vi "Drive Controller.vi"(8 "error in":errorcluster) -> ()   [LabVIEW 2017]
doc: "This VI executes continuously carrying out the current operation and responding to updates or new operation requests. It will often contain the timing or control code that is difficult to place directly in TeleOp. This VI generally opens all sensors and motors and isolates the rest of the robot code from knowing implementation details of how the operations are carried out."
uses:
  Drive Setpoints.ctl
  Drive Operations.ctl
  <vilib>/Rock Robotics/WPI/SafetyOutput/WPI_SafetyOutputConfigMenu.ctl
panel:
  out "error out":errorcluster
  in  "Control P":dbl=0.5
  out "Setpoints":T1(graph)
  out "Current\nCmd":string
  # "Tip: It may be helpful to observe inputs and sensor values.\nYou may also want to display tuning or debugging controls."
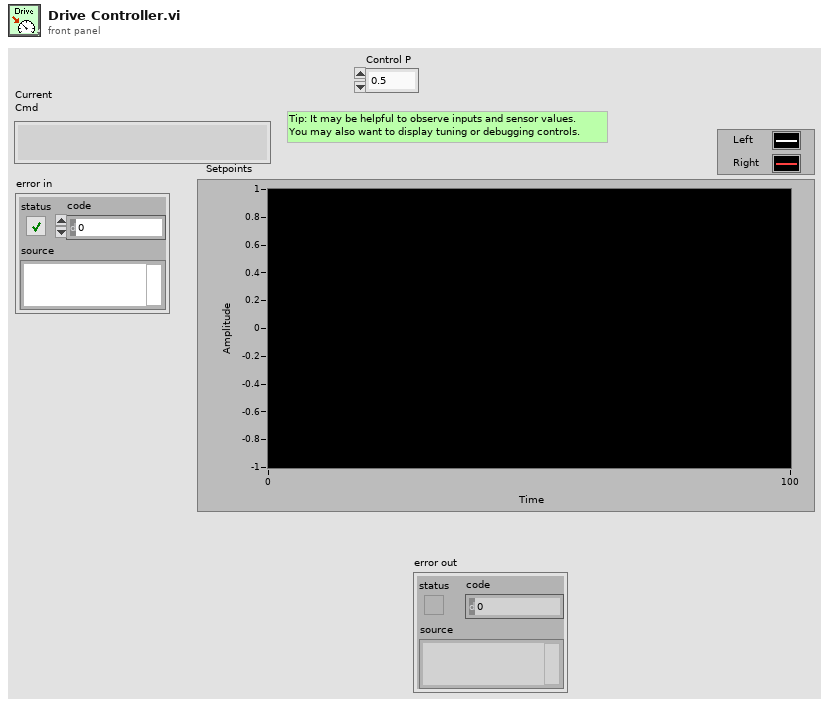
[diagram p1: front panel]
types:
  T1 = cluster{"Left Setpoint":dbl, "Right Setpoint":dbl}
  T2 = typedef "Drive Setpoints.ctl" = cluster{"Operation":T3, "Left Setpoint":dbl, "Right Setpoint":dbl, "Duration":dbl}
  T3 = typedef "Drive Operations.ctl" = enum16{"Reserve", "Read Current", "Immediate", "Drive for Time", "Drive for Distance"}
  T4 = typedef "WPI_SafetyOutputConfigMenu.ctl" = enum16{"Enable", "Disable"}
  T5 = typedef "WPI_RobotDriveDevRef.ctl" = cluster{"DevStatus":errorcluster, "Motors[]":T6[], "Square Inputs":bool, "Max Output":dbl}
  T6 = typedef "WPI_MotorControlDeviceRef.ctl" = cluster{"DeviceStatus":errorcluster, "Type":T7, "PWM":cluster{"PWM Channel":T8, "DeadBand":T9}, "CAN":cluster{"Device Number":u8, "SetOutput VI Ref":variant, "GetOutput VI Ref":variant, "Enable VI Ref":variant, "Disable VI Ref":variant, "Data":variant}, "Invert":bool, "DIO PWM":cluster{"PWM \"Enable\" Channel":T8, "DIOChannel":T10, "PWM Rate":dbl}}
  T7 = typedef "WPI_MotorControlType.ctl" = enum16{"PWM", "CAN", "DIO PWM"}
  T8 = typedef "FPGA_DIOPWMChannel.ctl" = enum8{"PWM 0", "PWM 1", "PWM 2", "PWM 3", "PWM 4", "PWM 5", "PWM 6", "PWM 7", "PWM 8", "PWM 9", "PWM MXP 0", "PWM MXP 1", "PWM MXP 2", "PWM MXP 3", "PWM MXP 4", "PWM MXP 5", "PWM MXP 6", "PWM MXP 7", "PWM MXP 8", "PWM MXP 9", "Invalid"}
  T9 = typedef "WPI_PWMDeadband.ctl" = cluster{"Name":string, "maxPositivePwm":i32, "minPositivePwm":i32, "centerPwm":i32, "maxNegativePwm":i32, "minNegativePwm":i32, "angularRange":u16}
  T10 = typedef "FPGA_DIOChannel.ctl" = enum8{"DIO 0", "DIO 1", "DIO 2", "DIO 3", "DIO 4", "DIO 5", "DIO 6", "DIO 7", "DIO 8", "DIO 9", "DIO MXP 0", "DIO MXP 1", "DIO MXP 2", "DIO MXP 3", "DIO MXP 4", "DIO MXP 5", "DIO MXP 6", "DIO MXP 7", "DIO MXP 8", "DIO MXP 9", "DIO MXP 10", "DIO MXP 11", "DIO MXP 12", "DIO MXP 13", "DIO MXP 14", "DIO MXP 15", "SPI Port CS1", "SPI Port CS2", "SPI Port CS3", "SPI Port MISO", "SPI Port MOSI", "Invalid"}
  T11 = typedef "Command Status Info.ctl" = cluster{"Name":string, "Status":T12, "notifier out":T13}
  T12 = typedef "Completion Status.ctl" = enum16{"Successful", "Aborted", "Incomplete"}
  T13 = typedef "Completion Notifier.ctl" = refnum<notifier>
  T14 = cluster{"SubSystem Data":T2, cluster{"Start Time (ms)":u32, "Iterations":i32}, cluster{"Command Info":T11, "Description":string, "SubSystem Data":T2, "notifier out":refnum<notifier>, "Subsystem Name":string}}
  T15 = cluster{"SubSystem Data":T2, cluster{"Start Time (ms)":u32, "Iterations":i32}, "Default Command Arguments":cluster{"Command Info":T11, "Description":string, "SubSystem Data":T2, "notifier out":refnum<notifier>, "Subsystem Name":string}}
  T16 = cluster{"Don't move motors while reserved":dbl, "Don't move motors while reserved":dbl}
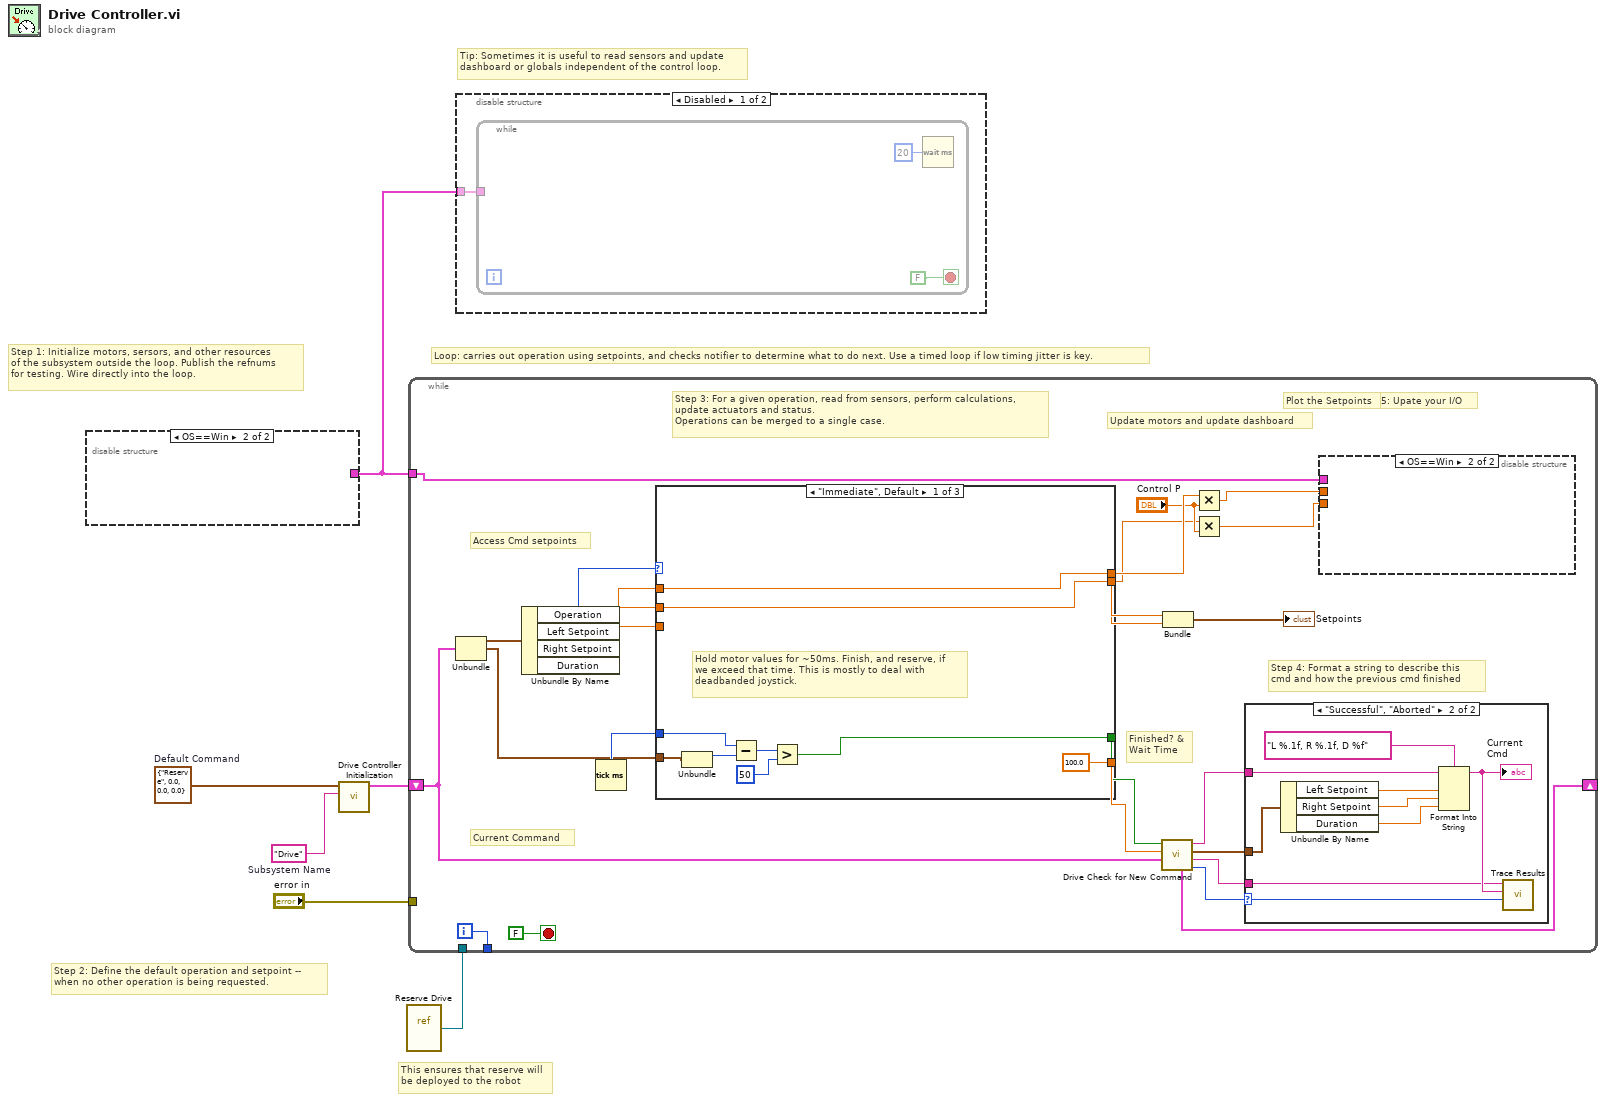
[diagram p0: block diagram]
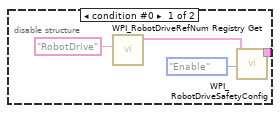
[diagram p2: hidden frame]
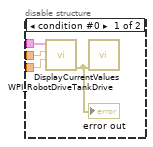
[diagram p4: hidden frame]
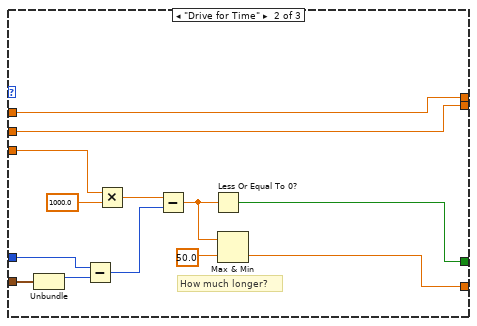
[diagram p6: hidden frame]
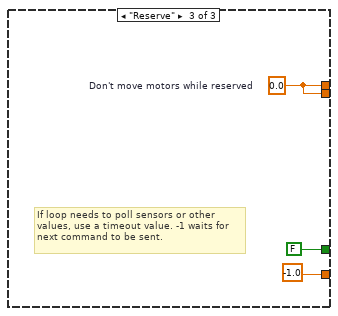
[diagram p7: hidden frame]
diagram:
  w5 = T2 {"Operation"=enum."Reserve", "Left Setpoint"=0.0, "Right Setpoint"=0.0, "Duration"=0.0}  # Default Command
  w6 = "Drive"  # Subsystem Name
  # "This ensures that reserve will\nbe deployed to the robot"
  # "Tip: Sometimes it is useful to read sensors and update\ndashboard or globals independent of the control loop."
  # "Step 2: Define the default operation and setpoint --\nwhen no other operation is being requested."
  # "Step 1: Initialize motors, sersors, and other resources\nof the subsystem outside the loop. Publish the refnums\nfor testing. Wire directly into the loop."
  # "Loop: carries out operation using setpoints, and checks notifier to determine what to do next. Use a timed loop if low timing jitter is key."
  n1 = disable-structure shown="OS==Win" {
    disable-tunnel: [w7 _] -> w4
    frame condition #0 {
      n2 = call <vilib>:"WPI_RobotDriveRefNum Registry Get.vi"("refnum name"="RobotDrive") -> ("RobotDriveDevRef"=w9:T5)  [unwired: 9 in, 1 out]
      n3 = call <vilib>:"WPI_RobotDriveSafetyConfig.vi"("mode"=WPI_SafetyOutputConfigMenu."Enable", "RobotDriveDevRef"=w9) -> ("RobotDriveDevRef"=w7:T5)  [unwired: 8 in, 1 out]
    }
    frame condition #1 (active) {
    }
  }
  n4 = call "Drive Controller Initialization.vi"("Subsystem Name"=w6, "Default Command"=w5) -> ("output cluster"=w2:T14)  [unwired: 9 in]
  n5 = vi-ref "Reserve Drive.vi"() -> (w1:refnum<vi>)
  n6 = while {
    shift-right: [w23] -> _
    shift-left: w2 -> [w16]
    tunnel: [w33] -> _
    tunnel: w4 -> [w31]
    tunnel: "error in" -> [_]
    tunnel: w1 -> [_]
    i -> [w33]
    stop <- FALSE stop-if-true
    # "Step 5: Upate your I/O"
    # "Step 4: Format a string to describe this\ncmd and how the previous cmd finished"
    # "Current Command"
    # "Update motors and update dashboard"
    # "Plot the Setpoints"
    # "Access Cmd setpoints"
    # "Finished? &\nWait Time"
    # "Step 3: For a given operation, read from sensors, perform calculations,\nupdate actuators and status.\nOperations can be merged to a single case."
    n7 = Unbundle(w16) -> ("SubSystem Data"=w30:T2, w17:cluster{"Start Time (ms)":u32, "Iterations":i32})  [unwired: 1 out]
    n8 = Unbundle By Name(w30) -> ("Operation"=w29:T3, "Left Setpoint"=w28:dbl, "Right Setpoint"=w27:dbl, "Duration"=w26:dbl)
    n9 = Tick Count (ms)() -> (millisecond timer value=w25:u32)
    n10 = case shown="\"Immediate\", Default" w29 {
      tunnel: [100.0 w57 -1.0] -> w22
      tunnel: [w49 w64 FALSE ("ignore previous (F)")] -> w21
      tunnel: w17 -> [w48 w66 _]
      tunnel: [w55 w63 w70] -> w15
      tunnel: [w54 w62 w70] -> w12
      tunnel: w28 -> [w55 w63 _]
      tunnel: w27 -> [w54 w62 _]
      tunnel: w26 -> [_ w61 _]
      tunnel: w25 -> [w50 w60 _]
      frame "Immediate", Default {
        # "Hold motor values for ~50ms. Finish, and reserve, if\nwe exceed that time. This is mostly to deal with\ndeadbanded joystick."
        n11 = Unbundle(w48) -> ("Start Time (ms)"=w51:u32)  [unwired: 1 out]
        n12 = Subtract(x=w50, y=w51) -> (x-y=w52:u32)
        n13 = Greater?(x=w52, y=u8 50 ("Left Motor")) -> (0:w49:bool)
      }
      frame "Drive for Time" {
        # "How much longer?"
        n14 = Unbundle(w66) -> ("Start Time (ms)"=w65:u32)  [unwired: 1 out]
        n15 = Subtract(x=w60, y=w65) -> (x-y=w69:u32)
        n16 = Multiply(x=w61, y=1000.0) -> (x*y=w68:dbl)
        n17 = Subtract(x=w68, y=w69) -> (x-y=w59:dbl)
        n18 = Less Or Equal To 0?(x=w59) -> (x <= 0?=w64:bool)
        n19 = Max & Min(x=w59, y=50.0) -> (min(x,y)=w57:dbl)  [unwired: 1 out]
      }
      frame "Reserve" {
        w70 = 0.0  # Don't move motors while reserved
        # "If loop needs to poll sensors or other\nvalues, use a timeout value. -1 waits for\nnext command to be sent."
      }
    }
    n20 = call "Drive Check for New Command.vi"("input cluster"=w16, "Wait time (ms)"=w22, "Finished?"=w21) -> ("Completion"=w24:T12, "Subsystem Name"=w18:string, "SetPoint"=w19:T2, "Initial Trace String"=w20:string, "output cluster"=w23:T15)  [unwired: 4 in]
    n21 = Bundle("Don't move motors while reserved"=w15, "Don't move motors while reserved"=w12) -> (→"Setpoints":T16)  [unwired: 1 in]
    n22 = Multiply(x=w15, y="Control P") -> (x*y=w14:dbl)
    n23 = Multiply(x=w12, y="Control P") -> (x*y=w11:dbl)
    n24 = case shown="\"Successful\", \"Aborted\"" w24 {
      selector: w24 -> [_ w47]
      tunnel: w20 -> [_ w42]
      tunnel: w19 -> [_ w43]
      tunnel: w18 -> [_ w39]
      frame "Incomplete", Default {
        # "Continuing current command"
      }
      frame "Successful", "Aborted" {
        # "Report and setup for next command"
        n25 = Unbundle By Name(w43) -> ("Left Setpoint"=w45:dbl, "Right Setpoint"=w46:dbl, "Duration"=w40:dbl)
        n26 = Format Into String(format string="L %.1f, R %.1f, D %f", initial string=w42, w45, w46, w40) -> (resulting string=w41:string)  [unwired: 1 in, 1 out]
        "Current\nCmd" <- w41
        n27 = call <vilib>:"Trace Results.vi"("Status of previous command"=w47, "Description"=w41, "Subsystem"=w39) -> ()  [unwired: 9 in]
      }
    }
    n28 = disable-structure shown="OS==Win" {
      disable-tunnel: w31 -> [w38 _]
      disable-tunnel: w14 -> [w37 _]
      disable-tunnel: w11 -> [w36 _]
      frame condition #0 {
        n29 = call <vilib>:"WPI_RobotDriveTankDrive.vi"("Right axis value"=w36, "Left axis value"=w37, "RobotDriveDevRef"=w38) -> ("error out"=w35:errorcluster)  [unwired: 6 in, 2 out]
        "error out" <- w35
        n30 = call "DisplayCurrentValues.vi"("error in (no error)"=w35) -> ()  [unwired: 6 in, 5 out]
      }
      frame condition #1 (active) {
      }
    }
  }
  n31 = disable-structure shown="Disabled" {
    disable-tunnel: w4 -> [w73 _]
    frame Disabled {
      n32 = while {
        tunnel: w73 -> [_]
        stop <- FALSE stop-if-true
        n33 = Wait (ms)(milliseconds to wait=u32 20) -> ()  [unwired: 1 out]
      }
    }
    frame Enabled {
    }
  }
